vi "CheckODEUserFunctionSignature.vi"(0 "Error Line Number in":u32, 1 "Function name":string, 5 "Error Column Number in":u32, 7 "MFilePath":path, 9 "MSCompiler Flags":T1, 11 "error in":errorcluster) -> (8 "error line nums out":u32[](array[numeric]), 10 "error col nums out":u32[](array[numeric]), 15 "Error outs":errorcluster[](array[cluster]))   [LabVIEW 2021]
uses:
  <vilib>/imath/engines/lvmath2/MathScriptCompiler/CTLs/NIMS_MSCompilerFlags.ctl
  <vilib>/imath/engines/lvmath/Functions/Error Handling/error.ctl
  <vilib>/imath/engines/lvmath2/MathScriptCompiler/MathScriptCompiler.llb/MathScriptCompiler.lvlib
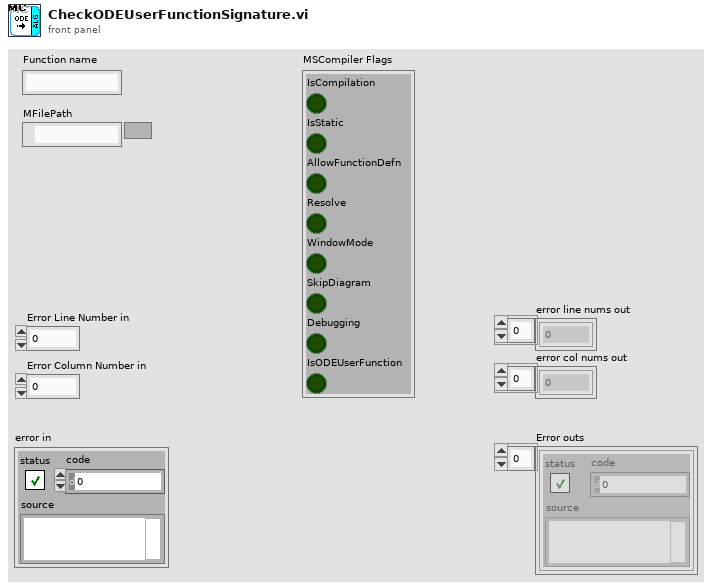
[diagram p1: front panel]
types:
  T1 = typedef "NIMS_MSCompilerFlags.ctl" = cluster{"IsCompilation":bool, "IsStatic":bool, "AllowFunctionDefn":bool, "Resolve":bool, "WindowMode":bool, "SkipDiagram":bool, "Debugging":bool, "IsODEUserFunction":bool}
  T2 = typedef "error.ctl" = enum16{"No Error", "Problem", "Input type must not be void", "Incorrect number of parameters", "Function not defined for non-numeric types", "An output variable of the user-defined function is undefined", "Function only defined for character arrays", "Function not defined for boolean, character, or single precision", "Function not defined for complex types", "Not a valid operation", "Inputs must be scalar", "Input matrices are not the same size", "Function only available on RT", "Input matrices must be nonnegative integers of the same type", "Arguments must be non-negative integers less than bitmax", "Number to complement must be less than 2^N", "Bit to get is outside range", "Bit to set is outside range", "Input must be real type ", "At least one parameter must be scalar", "Unable to display plug-in data on RT", "Function not defined for higher dimensional matrices", "Invalid attributes", "Wrong Type of Input Arguments", "Wrong Argument Option", "Invalid file identifier", "Indices must be real positive integers", "The variable is not a matrix data type.", "Number of elements must be the same for indices and values", "You cannot replace elements of a matrix with non-matrix data types.", "Cannot resize a 2D matrix with a linear index", "Unknown variable or symbol", "Indices out of range", "Empty matrix deletion can not be used with two indices", "Number of rows and columns must be the same for indices and values.", "Complex cannot be converted to Boolean", "Char cannot be converted to Boolean", "int64 cannot be converted to Boolean", "uint64 cannot be converted to Boolean", "You cannot convert a Boolean to a character.", "Incompatible input size in 3D surface function", "All rows must have the same number of columns", "Incompatible types", "Invalid matrix dimensions", "Dimension must be 1 or 2", "Base must be an integer between 2 and 36", "Invalid input", "Square matrix required", "Function 'timerstart' must be called before 'timerstop'", "Arguments must be positive real", "Step must not be zero", "Wrong number of input arguments", "Wrong number of output arguments", "Too many index arguments", "Input scalar must be >= 0", "Input scalar must be positive", "Input scalar must not be 0", "Input scalar must be in range [0,1]", "Can't use conditionally defined variable that's undefined", "Input must be a vector", "RT Exec Trace Toolkit not licensed", "Empty vector error", "All elements must be in domain [-1,1]", "All real elements of input vector must be >= 0", "All elements of input vector must be positive", "Values of input vectors are not compatible", "DAQmx not installed", "Input vector must be an increasing vector", "Dereferenced field does not exist within the struct", "A vector or matrix of structures must be indexed before it can be dereferenced", "Lenths of two input vectors are not compatible", "Invalid fieldname", "Empty matrix error", "Cannot use '.' on a type other than Struct", "Unused074", "Data type of the struct's field name is invalid", "Using . to dereference data that is not a struct", "Input struct contains invalid type ", "Size of input matrix is incompatible with input size", "Invalid format specifier", "Could not find field within struct", "Bad permutation array", "Mismatched fieldnames", "ode: User Function could not be opened", "ode: User Function signature does not meet ode requirements", "Unused085", "RunTime: MathScript could not be compiled", "Unknown function", "Only scalars and strings supported", "ode: User Function signature has incorrect number of inputs", "ode:User Function signature has incorrect number of outputs", "Range is too large", "End used without variable", "Function not available (RTE)", "Custom user error", "Arguments must be integers less than bitmax", "Shared library not found", "Header file not found", "Shared library already loaded", "Shared library not loaded", "Shared library function not found", "Shared library string return problem", "Problem calling shared library function", "Problem loading shared library from OS", "Problem parsing shared library header file", "Shared library incompatible types", "Shared library unsupported return type", "Shared library function not exported", "Shared library unsupported input type", "Problem unloading shared library from OS", "Function only available from UI", "Function specified in argument is missing", "An internal error has occurred", "Invalid object", "Invalid property", "Read-only property", "A break command has occurred", "A continue command has occurred", "A return command has occurred", "ode: times parameter invalid", "Function specified in argument has incorrect signature", "Function not found in file", "Reserved keyword cannot be defined as variable", "Reserved keyword cannot be defined as a function or script", "Arguments must be string literals", "Function not supported on this platform", "All columns must have the same number of rows", "Function ignored in RTE warning", "Cannot use : as a parameter that is not a variable", "Output can't be coerced to requested type", "Function not supported on current target", "Variable dependent on an unwired function input", "Unused132", "Unused133", "Unused134", "Unused135", "Unused136", "Unused137", "Unused138", "Unused139", "Global/Persistent must only take constants as arguments.", "Varargin must be last input in the function definition.", "Varargout must be last output in the function definition.", "Invalid output type. Cannot output a cell array of any type other than string.", "Invalid output type. Type is a dynamic struct.", "Invalid output type. Type is a struct that has a field whose type is not known until run-time", "Invalid output type. Type is a struct that has a field which is a plot object.", "MathScript parser DLL missing", "MathScript requires LabVIEW Full", "MathScript license is invalid or missing", "Varargout not supported except in assignments."}
  T3 = typedef "MC_UserFunction_UserFunctionSignature.ctl" = cluster{"LinkIdentity":string, "MFilePath":path, "InputVars":string[], "OutputVars":string[], "IsUserFunctionAScript?":bool, "SyntaxErrors?":bool, "Line number(s)":u32[], "Index(s)":u32[]}
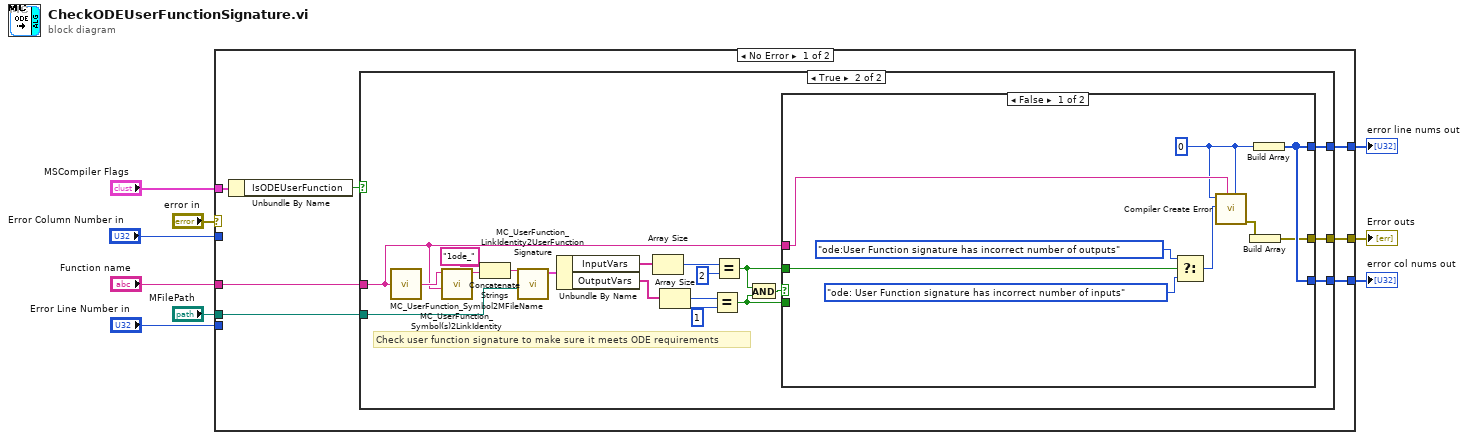
[diagram p0: block diagram]
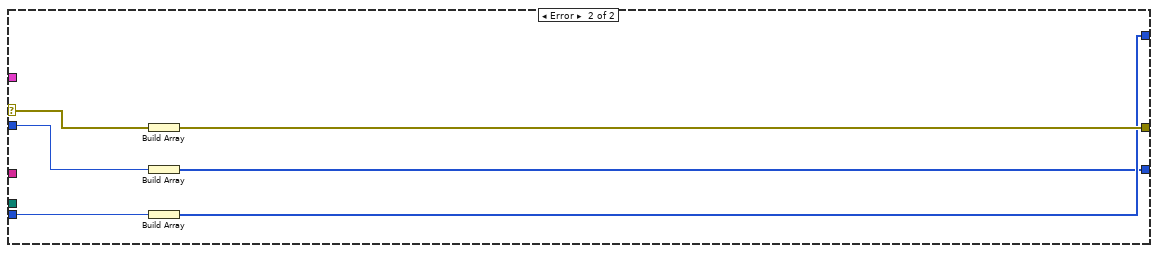
[diagram p4: hidden frame]
diagram:
  n1 = case shown="No Error" "error in" {
    selector: "error in" -> [_ w48]
    tunnel: "MFilePath" -> [w16 _]
    tunnel: "Function name" -> [w15 _]
    tunnel: [w14 w47] -> w7
    tunnel: "MSCompiler Flags" -> [w11 _]
    tunnel: [w13 w46] -> w5
    tunnel: [w12 w45] -> w4
    tunnel: "Error Column Number in" -> [_ w49]
    tunnel: "Error Line Number in" -> [_ w50]
    frame No Error {
      n2 = Unbundle By Name(w11) -> ("IsODEUserFunction"=w10:bool)
      n3 = case shown="True" w10 {
        tunnel: w16 -> [_ w34]
        tunnel: w15 -> [_ w20]
        tunnel: [_ w25] -> w14
        tunnel: [_ w24] -> w13
        tunnel: [_ w23] -> w12
        frame False {
        }
        frame True {
          # "Check user function signature to make sure it meets ODE requirements"
          n4 = call <vilib>:"MC_UserFunction_Symbol2MFileName.vi"("Symbol"=w20) -> ("MFileName"=w33:string)
          n5 = call <vilib>:"MC_UserFunction_Symbol(s)2LinkIdentity.vi"("FunctionName"=w20, "MFileName"=w33) -> ("LinkIdentity"=w18:string)  [unwired: 9 in]
          n6 = Concatenate Strings("1ode_" ("LinkIdentity"), w18) -> (w17:string)
          n7 = call <vilib>:"MC_UserFunction_LinkIdentity2UserFunctionSignature.vi"("MFilePath"=w34, "LinkIdentity"=w17) -> ("UserFunctionSignature out"=w32:T3)  [unwired: 8 in, 1 out]
          n8 = Unbundle By Name(w32) -> ("InputVars"=w28:string[], "OutputVars"=w27:string[])
          n9 = Array Size(array=w28) -> (size(s)=w26:i32)
          n10 = Array Size(array=w27) -> (size(s)=w30:i32)
          n11 = Equal?(x=w30, y=1) -> (x = y?=w21:bool)
          n12 = Equal?(x=w26, y=2 ("x")) -> (x = y?=w22:bool)
          n13 = And(x=w22, y=w21) -> (x .and. y?=w35:bool)
          n14 = case shown="False" w35 {
            tunnel: w20 -> [w44 _]
            tunnel: [w41 _] -> w24
            tunnel: [w41 _] -> w23
            tunnel: [w40 _] -> w25
            tunnel: w22 -> [w37 _]
            tunnel: w21 -> [_ _]
            frame False {
              w42 = u32 0 ("Line number")
              n15 = Select(t=error."ode:User Function signature has incorrect number of outputs" ("Error Enum"), s=w37, f=error."ode: User Function signature has incorrect number of inputs" ("Error Enum")) -> (s? t:f=w36:T2)
              n16 = call <vilib>:"Compiler Create Error.vi"("Column number"=w42, "Function name"=w44, "Error Enum"=w36, "Line number"=w42) -> ("error out"=w43:errorcluster)  [unwired: 7 in]
              n17 = Build Array(w43) -> (w40:errorcluster[])
              n18 = Build Array(w42) -> (w41:u32[])
            }
            frame True {
            }
          }
        }
      }
    }
    frame Error {
      n19 = Build Array(w48) -> (w47:errorcluster[])
      n20 = Build Array(w49) -> (w45:u32[])
      n21 = Build Array(w50) -> (w46:u32[])
    }
  }
  "error line nums out" <- w5
  "error col nums out" <- w4
  "Error outs" <- w7
